vi "Class - Controls.vi"(7 "Msg Chain":string, 8 "error in (no error)":errorcluster {"code" format="Error %.0f"}, 10 "Classes":refnum<class "Class Documentation.lvclass">[](array[class]), 11 "VIDoc Printer - Confluence In":refnum<class "VIDoc Printer - Confluence.lvclass">) -> (0 "error out":errorcluster {"code" format="Error %.0f"}, 3 "VIDoc Printer - Confluence Out":refnum<class "VIDoc Printer - Confluence.lvclass">)   [LabVIEW 2023, in "VIDoc Printer - Confluence.lvlib" / "VIDoc Printer - Confluence.lvclass"]
uses:
  VIDoc Printer - Confluence.lvclass
  C:/projects/DMC/GitHub/DMC CLI VIDoc/Source/Documentation Generation/Printers/Printer/VIDoc Printer.lvclass
  Parsing/Class Documentation/Class Documentation.lvclass
  Parsing/Class Documentation/Class Documentation.lvclass/Class Documentation.ctl
  Printer/VIDoc Printer.lvclass/VIDoc Printer.ctl
  Parsing/TypeDefs/VI Type Extended Enum.ctl
  Confluence Formatting/Types/Format Combo Box.ctl
  VIDoc Printer - Confluence.lvclass/VIDoc Printer - Confluence.ctl
  Accessors/Get Class Controls Expand.vi
  Printer/Accessors/Get Class Settings - Controls Detail Level.vi
  Printer/Accessors/Get Class Settings - Controls Scope.vi
  Parsing/Class Documentation/Get Methods.vi
  Parsing/Class Documentation/Get Name.vi
  Printer/VIDoc Printer.lvclass
  UI Interaction/UI Interaction.lvclass
  Parsing/VIDoc Parsing.lvlib
  Confluence Formatting/Confluence Formatting.lvlib
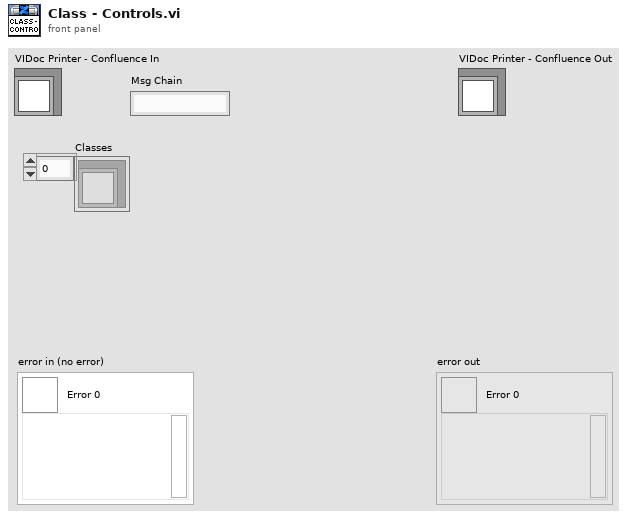
[diagram p1: front panel]
types:
  T1 = typedef "VIDoc Parsing.lvlib/VI Type Extended Enum.ctl" = enum16{"Unknown", "Class Method", "Class Accessor Get", "Class Accessor Set", "Class Control", "Library Method", "Library Control", "VI", "Control"}
  T2 = typedef "Confluence Formatting.lvlib/Format Combo Box.ctl" = string
  T3 = typedef "VIDoc Parsing.lvlib/Method Spec Cluster.ctl" = cluster{"VI Type Ext":T1, "Name":string, "Path":path, "Get Conpane Image":T4, "Description":string, "Get Library Access Scope":enum32{"invalid scope", "public", "private", "protected", "community"}, "Dispatch":T5, "ContainsCompiledCode":bool, "Exec.IsReentrant":bool, "Exec.ReentrancyType":enum16{"Share clones between instances", "Preallocate clone for each instance"}, "ExecInlining":bool, "ExecInlineIfPossible":bool, "Auto Err Handling":bool, "CodeComplexity":sgl, "Bookmark Tags":string[], "Control VI Type":enum32{"not a control VI", "control", "typedef", "strict typedef"}, "Controls":T6[], "VI Type":enum32{"invalid VI type", "Standard VI", "Control VI", "Global VI", "Polymorphic VI", "Configuration VI", "SubSystem", "Facade VI", "Method VI", "Statechart Diagram VI"}, "Minimum Size":T8, "Front Panel Window:Title":string, "Front Panel Window:Behavior":enum32{"Invalid", "Default", "Floating", "Floating/Auto-Hide", "Modal"}, "Front Panel Window:Closeable":bool, "Must Override":bool, "Must Use Parent Implementation":bool, "VI Icon":T4, "Front Panel":T4, "History:Revision Number":u32, "Metrics:Total Data Size":u32, "Execution:Allow Debugging":bool, "Execution:Preferred Exec System":enum32{"invalid execution system", "user interface", "standard", "instrument i/o", "data acquisition", "other 1", "other 2", "same as caller"}, "Execution:Priority":enum32{"invalid priority", "background priority", "normal priority", "above normal priority", "high priority", "time critical priority", "subroutine"}, "BM Tag Text":string[], "Block Diagram":T4, "Structure Tree":T9[]}
  T4 = typedef "imagedata.ctl" = cluster{"image type":i32, "image depth":i32, "image":u8[], "mask":u8[], "colors":u32[], "Rectangle":cluster{"left":i16, "top":i16, "right":i16, "bottom":i16}}
  T5 = typedef "VIDoc Parsing.lvlib/Class Dispatch Type Enum.ctl" = enum16{"None", "Static", "Dynamic"}
  T6 = typedef "VIDoc Parsing.lvlib/Controls Info Cluster.ctl" = cluster{"Name":string, "Description":string, "Data Type":string, "Tip Strip":string, "UID":i32, "Image Data":T4, "ToggleKeyBind":T7, "Raw Label":string, "Raw Caption":string}
  T7 = typedef "LVKeyTypeDef.ctl" = cluster{"Focus":bool, "Control":bool, "Shift":bool, "Key":string}
  T8 = typedef "LVPointTypeDef.ctl" = cluster{"Horizontal":i16, "Vertical":i16}
  T9 = typedef "VIDoc Parsing.lvlib/Structure Reporter.lvlib/Tree Cluster.ctl" = cluster{"Object Class Name":string, "Labels":string[], "Child Tag":string, "Item Indent":i32, "Child Only?":bool, "Glyph Index":i32}
  T10 = typedef "VIDoc Printer.lvlib/Printer Settings.lvclass/Detail Level Enum.ctl" = enum16{"None", "Minimal", "Standard", "Full"}
  T11 = typedef "VIDoc Printer.lvlib/Printer Settings.lvclass/Scope Settings.ctl" = cluster{"Public":bool, "Protected":bool, "Community":bool, "Private":bool, "Unknown":bool}
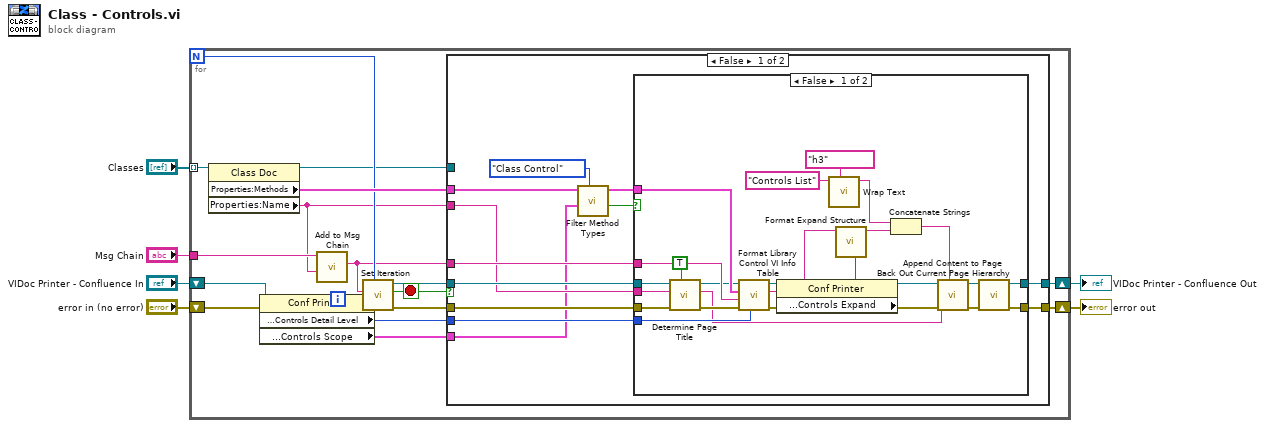
[diagram p0: block diagram]
diagram:
  n1 = for {
    N -> [w18]
    shift-right: [w23] -> w6
    shift-left: "error in (no error)" -> [w21]
    shift-right: [w24] -> w5
    shift-left: "VIDoc Printer - Confluence In" -> [w11]
    tunnel: "Classes" -> [w25] mode=indexing
    tunnel: "Msg Chain" -> [w16]
    i -> [w17]
    stop <- w14 stop-if-true
    n2 = property class="Class Doc"(reference=w25) -> (reference out=w13:refnum<class "Class Documentation.lvclass">, "Properties:Methods"=w22:T3[], "Properties:Name"=w15:string)  [unwired: 1 in, 1 out]
    n3 = property class="Conf Printer"(reference=w11, error in=w21) -> (reference out=w10:refnum<class "VIDoc Printer - Confluence.lvclass">, error out=w12:errorcluster, "Properties:Settings:Classes:Controls Detail Level"=w8:T10, "Properties:Settings:Classes:Controls Scope"=w7:T11)
    n4 = call "Add to Msg Chain.vi"("New"=w15, "Msg Chain in"=w16) -> ("Msg Chain out"=w9:string)  [unwired: 9 in]
    n5 = call "Set Iteration.vi"("Progress Max"=w18, "error in (no error)"=w12, "Progress Value"=w17, "Message (No Message Update)"=w9, "VIDoc Printer In"=w10) -> ("error out"=w19:errorcluster, "Abort?"=w14:bool, "VIDoc Printer Out"=w20:refnum<class "VIDoc Printer - Confluence.lvclass">)  [unwired: 4 in]
    n6 = case shown="False" w14 {
      tunnel: [w37 w64] -> w24
      tunnel: [w36 w65] -> w23
      tunnel: w22 -> [w32 _]
      tunnel: w20 -> [w34 w64]
      tunnel: w19 -> [w35 w65]
      tunnel: w15 -> [w30 _]
      tunnel: w13 -> [_ _]
      tunnel: w9 -> [w33 _]
      tunnel: w8 -> [w29 _]
      tunnel: w7 -> [w28 _]
      frame False {
        n7 = call "Filter Method Types.vi"("VI Type to filter for"=VI_Type_Extended_Enum."Class Control" ("y"), "Scope"=w28, "Methods"=w32) -> ("All Filtered?"=w26:bool, "Filtered Methods"=w31:T3[])  [unwired: 6 in, 1 out]
        n8 = case shown="False" w26 {
          tunnel: [w48 w63] -> w37
          tunnel: [w50 w62] -> w36
          tunnel: w35 -> [w46 w62]
          tunnel: w34 -> [w47 w63]
          tunnel: w33 -> [w54 _]
          tunnel: w29 -> [w53 _]
          tunnel: w31 -> [w51 _]
          tunnel: w30 -> [w41 _]
          frame False {
            n9 = call "Determine Page Title.vi"("Update Current Page (F)"=TRUE, "error in (no error)"=w46, "Name"=w41, "VIDoc Printer - Confluence In"=w47) -> ("error out"=w44:errorcluster, "Page Title"=w42:string, "VIDoc Printer - Confluence Out"=w45:refnum<class "VIDoc Printer - Confluence.lvclass">)  [unwired: 4 in, 1 out]
            n10 = call "Format Library Control VI Info Table.vi"("Methods"=w53, "Error in"=w44, "Msg Chain"=w54, "VI Info Array"=w51, "VIDoc Printer - Confluence In"=w45) -> ("Error out"=w56:errorcluster, "Table String"=w52:string, "VIDoc Printer - Confluence Out"=w55:refnum<class "VIDoc Printer - Confluence.lvclass">)  [unwired: 4 in]
            n11 = property class="Conf Printer"(reference=w55) -> (reference out=w39:refnum<class "VIDoc Printer - Confluence.lvclass">, "Properties:Expand?:Class:Controls Expand"=w38:bool)  [unwired: 1 in, 1 out]
            n12 = call "Wrap Text.vi"("Formatting"=T2 "h3", "String"="Controls List") -> ("Wrapped String"=w58:string)  [unwired: 8 in, 1 out]
            n13 = call "Format Expand Structure.vi"("Enable? (T)"=w38, "Content"=w52) -> ("Expand String"=w40:string)  [unwired: 8 in, 1 out]
            n14 = Concatenate Strings(w58, w40) -> (w57:string)
            n15 = call "Append Content to Page.vi"("Page Content"=w57, "error in (no error)"=w56, "Page Title"=w42, "VIDoc Printer - Confluence In"=w39) -> ("error out"=w61:errorcluster, "VIDoc Printer - Confluence Out"=w49:refnum<class "VIDoc Printer - Confluence.lvclass">)  [unwired: 6 in]
            n16 = call "Back Out Current Page Hierarchy.vi"("error in (no error)"=w61, "VIDoc Printer - Confluence In"=w49) -> ("error out"=w50:errorcluster, "VIDoc Printer - Confluence Out"=w48:refnum<class "VIDoc Printer - Confluence.lvclass">)  [unwired: 8 in]
          }
          frame True {
          }
        }
      }
      frame True {
      }
    }
  }
  "error out" <- w6
  "VIDoc Printer - Confluence Out" <- w5
